vi "Start_Task.vi"() -> (2 "QueueName":string)   [LabVIEW 2024]
doc: "Funkcja służy do inicjalizacji VI deamona piekarnika, generuje dedykowaną kolejkę do komunikacji pomiędzy główną aplikacją, a wątkiem deamona."
uses:
  <vilib>/numeric/Random Number (Range) U64.vi
  <vilib>/numeric/sub_Random U32.vi
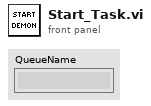
[diagram p1: front panel]
types:
  T1 = enum32{"Bad", "Idle", "Run top level", "Running"}
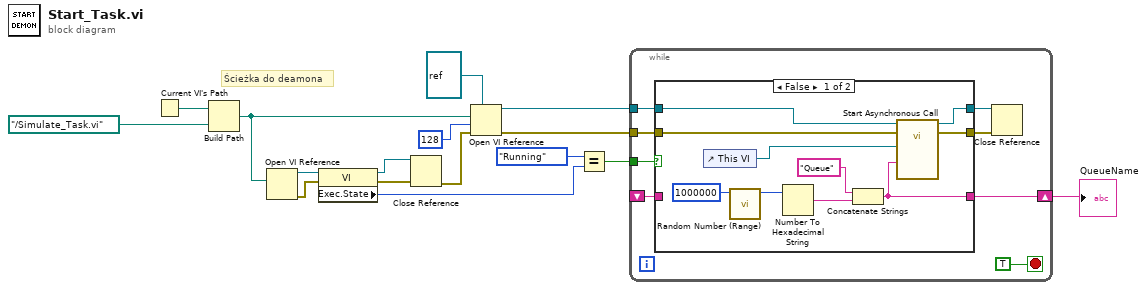
[diagram p0: block diagram]
diagram:
  # "Ścieżka do deamona"
  n1 = Current VI's Path() -> (path=w16:path)
  n2 = Build Path(base path=w16, name or relative path=path "../Simulate_Task.vi" ("vi path")) -> (appended path=w10:path)
  n3 = Open VI Reference(vi path=w10) -> (vi reference=w9:refnum<vi>, error out=w6:errorcluster)  [unwired: 5 in]
  n4 = property class="VI"(reference=w9, error in=w6) -> (reference out=w5:refnum<vi>, error out=w3:errorcluster, "Exec.State"=w4:T1)
  n5 = Close Reference(reference=w5, error in (no error)=w3) -> (error out=w2:errorcluster)
  n6 = Open VI Reference(type specifier VI Refnum (for type only)=refnum<vi> refnum, vi path=w10, options=128, error in (no error)=w2) -> (vi reference=w12:refnum<vi>, error out=w7:errorcluster)  [unwired: 2 in]
  n7 = Equal?(x=T1."Running", y=w4) -> (x = y?=w8:bool)
  n8 = while {
    tunnel: w12 -> [w24]
    tunnel: w8 -> [w23]
    tunnel: w7 -> [w22]
    shift-right: [w18] -> w1
    shift-left: _ -> [w17]
    stop <- TRUE stop-if-true
    n9 = case shown="False" w23 {
      tunnel: w24 -> [w34 w37]
      tunnel: w22 -> [w32 w36]
      tunnel: [w31 w36] -> w21
      tunnel: [w30 w37] -> w20
      tunnel: [w25 w35] -> w18
      tunnel: w17 -> [_ w35]
      frame False {
        n10 = control-ref of="This VI"() -> (w33:refnum<vi>)
        n11 = call-poly <vilib>:"Random Number (Range).vi"("upper bound (100)"=u64 1000000) -> ("number"=w28:u64)  [unwired: 10 in]
        n12 = Number To Hexadecimal String(2:w28) -> (0:w27:string)  [unwired: 1 in]
        n13 = Concatenate Strings("Queue" ("string"), w27) -> (w25:string)
        n14 = call-by-ref "Start Asynchronous Call"(reference=w34, error in=w32, "DeamonQueueName"=w25, "Parent VI"=w33) -> (reference out=w30:refnum<vi>, error out=w31:errorcluster)  [unwired: 10 in]
      }
      frame True {
      }
    }
    n15 = Close Reference(reference=w20, error in (no error)=w21) -> ()  [unwired: 1 out]
  }
  "QueueName" <- w1
